vi "GetVIItemIDs.vi"(8 "error in (no error)":errorcluster, 11 "BaseAccessorScripter in":refnum<class "BaseAccessorScripter.lvclass">) -> (0 "error out":errorcluster, 2 "VI ItemIDs":string[](array[string]), 3 "BaseAccessorScripter out":refnum<class "BaseAccessorScripter.lvclass">)   [LabVIEW 2021, in "MemberVICreation.lvlib" / "BaseAccessorScripter.lvclass"]
uses:
  <resource>/Framework/Providers/LVClassLibrary/NewAccessors/BaseAccessorScripter/BaseAccessorScripter.lvclass
  <resource>/Framework/Providers/LVClassLibrary/NewAccessors/BaseAccessorScripter/BaseAccessorScripter.lvclass/BaseAccessorScripter.ctl
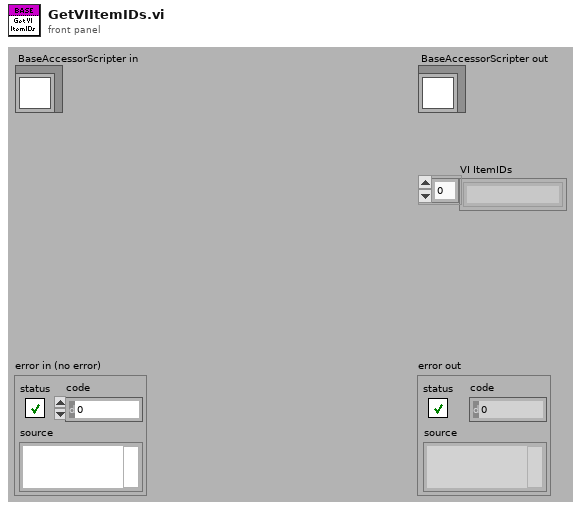
[diagram p1: front panel]
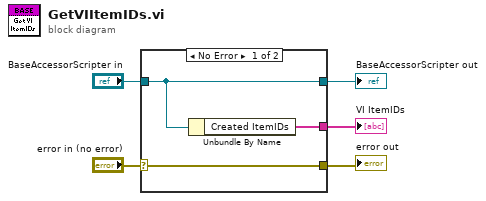
[diagram p0: block diagram]
diagram:
  n1 = case shown="No Error" "error in (no error)" {
    selector: "error in (no error)" -> [w8 w10]
    tunnel: [w8 w10] -> w4
    tunnel: [w7 w9] -> w2
    tunnel: "BaseAccessorScripter in" -> [w7 w9]
    tunnel: [w6 _] -> w1
    frame No Error {
      n2 = Unbundle By Name(w7) -> ("Created ItemIDs"=w6:string[])
    }
    frame Error {
    }
  }
  "error out" <- w4
  "BaseAccessorScripter out" <- w2
  "VI ItemIDs" <- w1
